vi "Insert Into SubPanel.vi"(8 "error in (no error)":errorcluster caption="Error In", 9 "SubPanel Ref":refnum<vi>, 10 "VI Path":path, 11 "VI Ref In":refnum<vi>) -> (0 "error out":errorcluster caption="Error Out")   [LabVIEW 2020]
panel:
  # "传入VI的引用或者VI路径程序都可以自动判断"
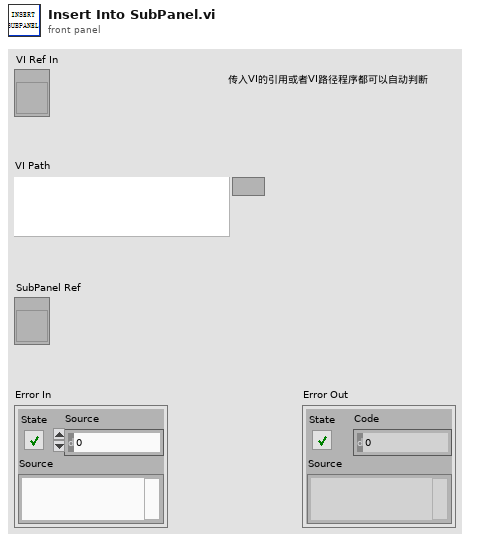
[diagram p1: front panel]
types:
  T1 = enum32{"Invalid", "Standard", "Closed", "Hidden", "Minimized", "Maximized"}
  T2 = enum32{"Bad", "Idle", "Run top level", "Running"}
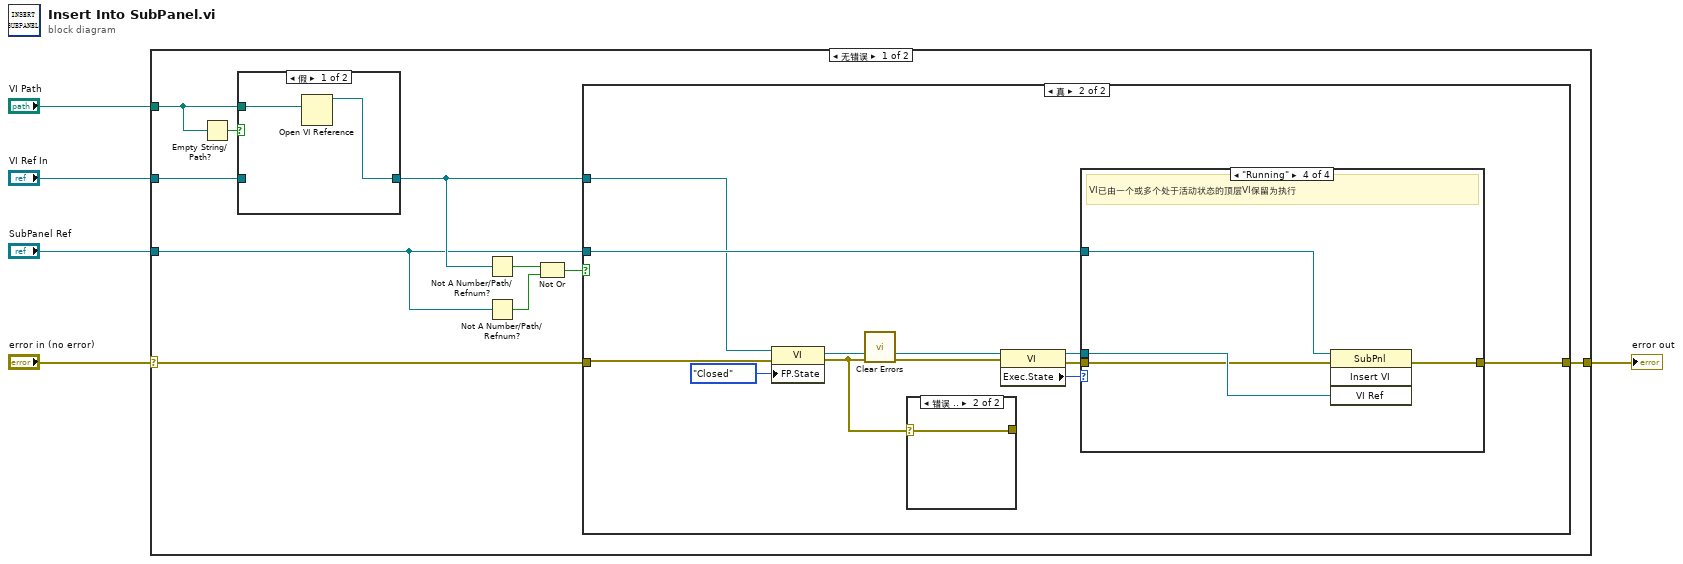
[diagram p0: block diagram]
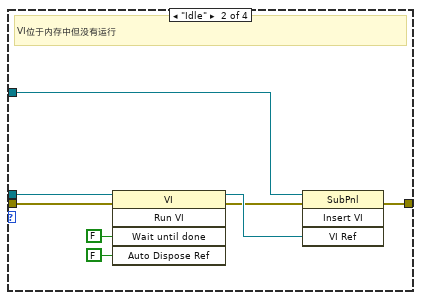
[diagram p5: hidden frame]
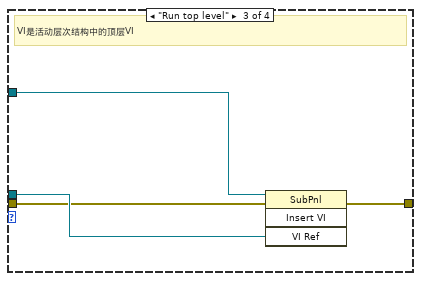
[diagram p6: hidden frame]
diagram:
  n1 = case shown="无错误" "error in (no error)" {
    selector: "error in (no error)" -> [w15 w49]
    tunnel: [w14 w49] -> w4
    tunnel: "VI Path" -> [w13 _]
    tunnel: "SubPanel Ref" -> [w9 _]
    tunnel: "VI Ref In" -> [w11 _]
    frame No Error {
      n2 = Empty String/Path?(string/path=w13) -> (empty?=w12:bool)
      n3 = case shown="假" w12 {
        tunnel: w13 -> [w47 _]
        tunnel: [w46 w48] -> w10
        tunnel: w11 -> [_ w48]
        frame False {
          n4 = Open VI Reference(vi path=w47) -> (vi reference=w46:refnum<vi>)  [unwired: 5 in, 1 out]
        }
        frame True {
        }
      }
      n5 = Not A Number/Path/Refnum?(number/path/refnum=w10) -> (NaN/Path/Refnum?=w7:bool)
      n6 = Not A Number/Path/Refnum?(number/path/refnum=w9) -> (NaN/Path/Refnum?=w8:bool)
      n7 = Not Or(1:w8, 2:w7) -> (0:w6:bool)
      n8 = case shown="真" w6 {
        tunnel: w15 -> [w16 w21]
        tunnel: [w16 w27] -> w14
        tunnel: w9 -> [_ w26]
        tunnel: w10 -> [_ w20]
        frame False {
        }
        frame True {
          n9 = property class="VI"(reference=w20, error in=w21, "FP.State"=T1."Closed" ("前面板窗口:状态")) -> (reference out=w18:refnum<vi>, error out=w17:errorcluster)
          n10 = call <vilib>:"Clear Errors.vi"("error in (no error)"=w17) -> ("error out"=w19:errorcluster)  [unwired: 5 in, 1 out]
          n11 = case shown="错误 .." w17 {
            selector: w17 -> [_ w28]
            tunnel: [_ w28] -> _
            frame No Error {
            }
            frame Error {
            }
          }
          n12 = property class="VI"(reference=w18, error in=w19) -> (reference out=w24:refnum<vi>, error out=w23:errorcluster, "Exec.State"=w25:T2)
          n13 = case shown="\"Running\"" w25 {
            tunnel: w24 -> [_ w37 w41 w44]
            tunnel: w26 -> [_ w34 w40 w45]
            tunnel: w23 -> [w29 w32 w38 w42]
            tunnel: [w29 w30 w39 w43] -> w27
            frame "Bad", Default {
              # "VI包含错误并且无法执行。"
            }
            frame "Idle" {
              # "VI位于内存中但没有运行"
              n14 = invoke class="VI" method="Run VI"(reference=w37, error in=w32, "Wait until done"=FALSE ("结束前等待"), "Auto Dispose Ref"=FALSE ("自动销毁引用")) -> (reference out=w33:refnum<vi>, error out=w31:errorcluster)  [unwired: 1 in, 3 out]
              n15 = invoke class="SubPnl" method="Insert VI"(reference=w34, error in=w31, "VI Ref"=w33) -> (error out=w30:errorcluster)  [unwired: 1 in, 3 out]
            }
            frame "Run top level" {
              # "VI是活动层次结构中的顶层VI"
              n16 = invoke class="SubPnl" method="Insert VI"(reference=w40, error in=w38, "VI Ref"=w41) -> (error out=w39:errorcluster)  [unwired: 1 in, 3 out]
            }
            frame "Running" {
              # "VI已由一个或多个处于活动状态的顶层VI保留为执行"
              n17 = invoke class="SubPnl" method="Insert VI"(reference=w45, error in=w42, "VI Ref"=w44) -> (error out=w43:errorcluster)  [unwired: 1 in, 3 out]
            }
          }
        }
      }
    }
    frame Error {
    }
  }
  "error out" <- w4
